vi "Komponentenausgabe.vi"(8 "error in (no error)":errorcluster caption="Fehler (Eingang, kein Fehler)") -> (0 "error out":errorcluster caption="Fehler (Ausgang)", 1 "Gasnummer out":u8, 2 "Konzentration":sgl, 3 "Gaskomponente":T1)   [LabVIEW 2020, in "Linearisierung v2.lvlib"]
uses:
  Linearisierung v2.lvlib
  Visualisierungs Elemente/Auswahlfeld.ctl
  Aktion Lin Daten aufarbeiten.ctl
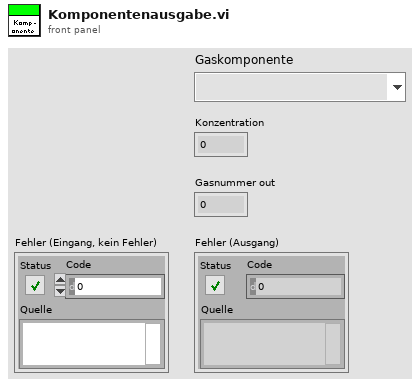
[diagram p1: front panel]
types:
  T1 = typedef "Auswahlfeld.ctl" = u16
  T2 = typedef "Linearisierung v2.lvlib/Aktion Lin Daten aufarbeiten.ctl" = enum16{"lesen", "Protkolldaten", "speichern", "laden", "EPA auswerten", "Tabelle schreiben", "Lin auswerten", "Tab init", "Stufentabelle", "EPA aktiviert", "Nachbehandlung laden", "Tabelle löschen", "Istwerte löschen", "Zeile löschen", "Zeile einfügen", "LIN aktiviert", "LIN/EPA aktiv laden", "EGAK Tab", "LIN übernehmen", "Tab init ohne Stufen"}
  T3 = typedef "Linearisierung v2.lvlib/Lin-Polynom Daten.ctl" = cluster{"Messgerät":string, "Kalibrator (Gasteiler)":string, "Bearbeiter/in":string, "Komponente":string, "Zeitstempel":timestamp, "F_max gefordert (%)":sgl, "F_max in %":sgl, "F_max in ppm":sgl, "Vorschlag Ordnung":i32, "Polynom OK":bool, "Polynomkoeff.":dbl[], "Prüfgas Konzentration":dbl, "Pfad EPA":string, "Pfad_LIN":string, "Gasnummer:":u8, "Komponentenauswahl":T4, "Verdünnungsgas":T5, "Zeitdauer Stufe":T6, "Anzahl Stufen":T6, "F_max in % EPA":sgl, "F_max in ppm EPA":sgl, "F_max in % LIN":sgl, "F_max in ppm LIN":sgl, "Punkte umkehren":bool, "EPA Optionsfeld":T7, "Autolin Hovacal":T8, "Spanfactors":sgl[], "Kalibrierauswahl":T9, "Conditions:":T10, "Gasflaschen Nr.:":string, "Bottle Accuracy":dbl, "Konfig Gasflasche":T11, "Gasflasche":T12, "HovaCAL Flow AutoLin":T13, "MFC Output":T14, "Gas Ablaufdatum":timestamp, "Lin Modus":T15, "zusätzliche Zeitdauer Erster Punkt":sgl, "Offsets":sgl[]}
  T4 = typedef "Linearisierung v2.lvlib/KomponentenArray.ctl" = cluster{"Komponente:":T1, "Konzentration":dbl}[]
  T5 = typedef "Linearisierung v2.lvlib/Gasteiler.lvlib/Prüfgas in.ctl" = u16
  T6 = typedef "Zahlen-Eingabefeld.ctl" = sgl
  T7 = typedef "Linearisierung v2.lvlib/EPA Optionsfeld.ctl" = enum32{"Istwert", "Rohwert", "Linearisierter Wert"}
  T8 = typedef "Linearisierung v2.lvlib/Gasteiler.lvlib/HovaCal.lvlib/AutoLin Hovacal.ctl" = enum32{"Keine Auswahl", "Optionsauswahl 1", "Optionsauswahl 2"}
  T9 = typedef "Linearisierung v2.lvlib/Kalibrieroption.ctl" = u16
  T10 = typedef "Linearisierung v2.lvlib/Linearity verification 1065-307.lvlib/Condition.ctl" = u16
  T11 = typedef "System Einstellungen V2.lvlib/Konfig Gasflasche.ctl" = bool
  T12 = typedef "System Einstellungen V2.lvlib/Gasflasche Auswahl.ctl" = u16
  T13 = typedef "Linearisierung v2.lvlib/Gasteiler.lvlib/HovaCAL_Interface.lvlib/Controls.lvlib/Flow Einstellung.ctl" = cluster{"HovaCAL Flow Input Cluster":dbl}
  T14 = typedef "Linearisierung v2.lvlib/Gasteiler.lvlib/HovaCAL_Interface.lvlib/Controls.lvlib/Pump state.ctl" = cluster{"Run":bool}
  T15 = typedef "CalGas Aufschaltung.lvlib/Lin Modus.ctl" = u16
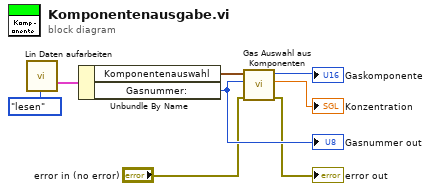
[diagram p0: block diagram]
diagram:
  n1 = call "Lin Daten aufarbeiten.vi"("Aktionen"=Aktion_Lin_Daten_aufarbeiten."lesen") -> ("Lin-Polynom"=w7:T3)  [unwired: 16 in, 10 out]
  n2 = Unbundle By Name(w7) -> ("Komponentenauswahl"=w6:T4, "Gasnummer:"=w5:u8)
  "Gasnummer out" <- w5
  n3 = call "Gas Auswahl aus Komponenten.vi"("Fehler (Eingang, kein Fehler)"="error in (no error)", "Gasnummer:"=w5, "Komponentenauswahl"=w6) -> ("Fehler (Ausgang)"=→"error out":errorcluster, "Konzentration"=→"Konzentration":dbl, "Auswahl"=→"Gaskomponente":T1)  [unwired: 6 in]
